vi "Zadanie 2.vi"() -> ()   [LabVIEW 2020]
panel:
  out "~Q":bool
  out "Q":bool
  in  "R":bool
  in  "C":bool
  in  "D":bool
  out "~Q":bool
  out "Q":bool
  in  "R":bool
  in  "K":bool
  in  "C":bool
  in  "J":bool
  out "~Q":bool
  out "Q":bool
  in  "R":bool
  in  "S":bool
  in  "Don't stop me now":bool
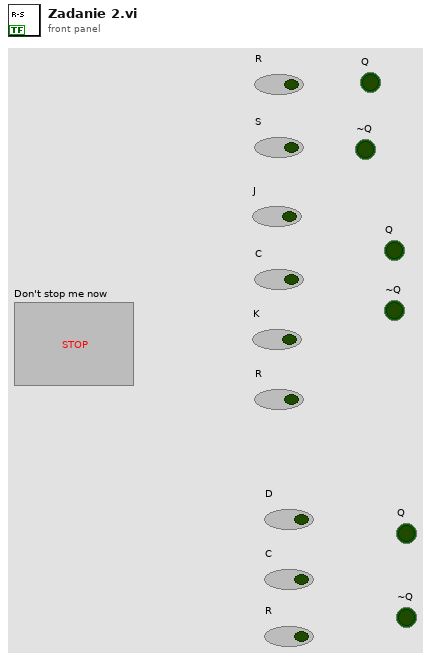
[diagram p1: front panel]
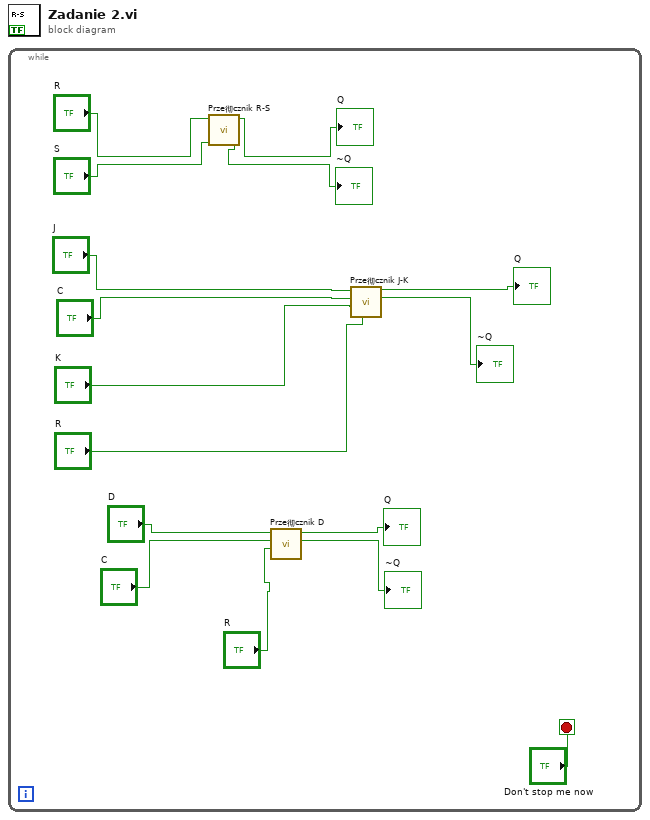
[diagram p0: block diagram]
diagram:
  n1 = while {
    stop <- "Don't stop me now" stop-if-true
    n2 = call "Prze彻cznik R-S.vi"("S"="S", "R"="R") -> ("~Q"=→"~Q":bool, "Q"=→"Q":bool)  [unwired: 8 in]
    n3 = call "Prze彻cznik D.vi"("R"="R", "C"="C", "D"="D") -> ("~Q"=→"~Q":bool, "Q"=→"Q":bool)  [unwired: 7 in]
    n4 = call "Prze彻cznik J-K.vi"("R"="R", "K"="K", "C"="C", "J"="J") -> ("~Q"=→"~Q":bool, "Q"=→"Q":bool)  [unwired: 6 in]
  }
